vi "FORMAS DE GUARDADO.vi"   [LabVIEW 2019]
uses:
  <vilib>/Utility/file.llb/Write Delimited Spreadsheet (DBL).vi
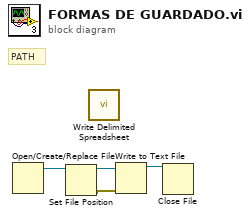
[diagram p0: block diagram]
diagram:
  # "PATH"
  n1 = Open/Create/Replace File() -> (refnum out=w3:refnum<file>)  [unwired: 6 in, 2 out]
  n2 = Set File Position(refnum=w3) -> (refnum out=w2:refnum<file>, error out=w4:errorcluster)  [unwired: 3 in]
  n3 = call-poly <vilib>:"Write Delimited Spreadsheet.vi"() -> ()  [unwired: 14 in, 2 out]
  n4 = Write to Text File(file (use dialog)=w2, error in=w4) -> (refnum out=w1:refnum<file>)  [unwired: 2 in, 2 out]
  n5 = Close File(refnum=w1) -> ()  [unwired: 1 in, 2 out]
